vi "Verify Idle.vi"(8 "error in (no error)":errorcluster, 11 "Instrument in":refnum<class "Instrument.lvclass">) -> (0 "error out":errorcluster, 3 "Instrument out":refnum<class "Instrument.lvclass">)   [LabVIEW 2018, in "Instrument.lvclass"]
uses:
  Instrument.lvclass
  Instrument.lvclass/Instrument.ctl
  Device/Optics/Opt_Selector/Opt_Selector.lvclass
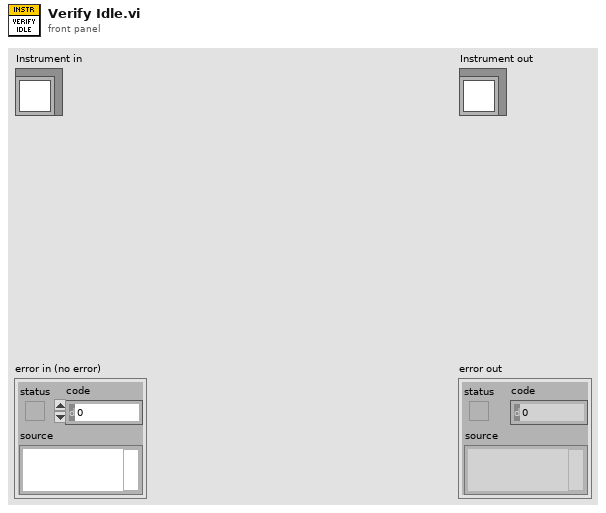
[diagram p1: front panel]
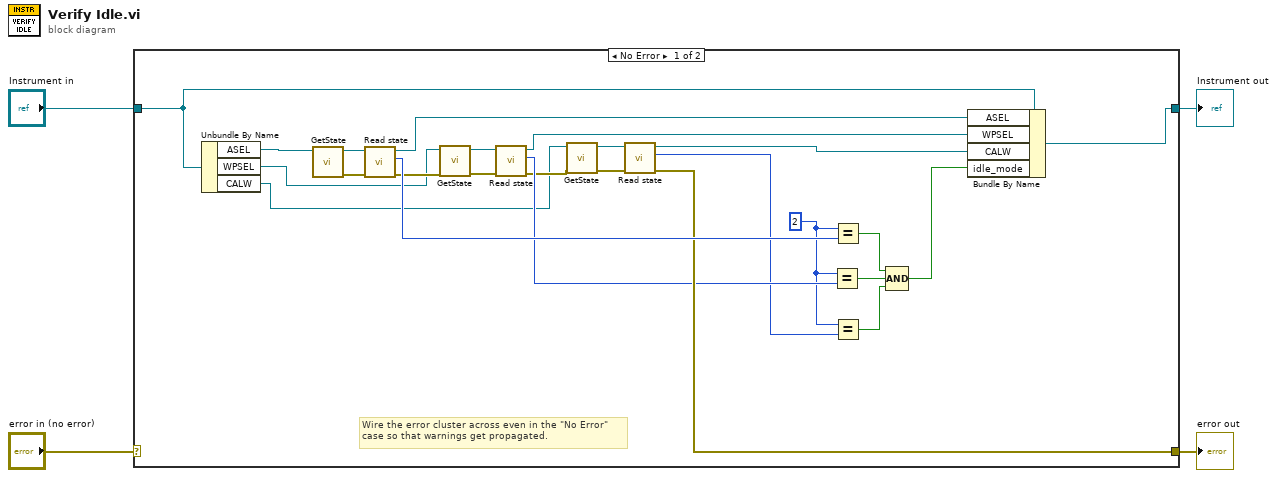
[diagram p0: block diagram]
diagram:
  n1 = case shown="No Error" "error in (no error)" {
    selector: "error in (no error)" -> [_ w31]
    tunnel: [w22 w31] -> w3
    tunnel: [w6 w30] -> w1
    tunnel: "Instrument in" -> [w10 w30]
    frame No Error {
      w19 = 2
      # "Wire the error cluster across even in the \"No Error\"\ncase so that warnings get propagated."
      n2 = Unbundle By Name(w10) -> ("ASEL"=w15:refnum<class "Opt_Selector.lvclass">, "WPSEL"=w12:refnum<class "Opt_Selector.lvclass">, "CALW"=w11:refnum<class "Opt_Selector.lvclass">)
      n3 = call-dynamic "GetState.vi"("Optics in"=w15) -> ("error out"=w28:errorcluster, "Optics out"=w29:refnum<class "Opt_Selector.lvclass">)  [unwired: 9 in]
      n4 = call-dynamic "Read state.vi"("error in (no error)"=w28, "Optics in"=w29) -> ("error out"=w14:errorcluster, "state"=w25:u8, "Optics out"=w9:refnum<class "Opt_Selector.lvclass">)  [unwired: 7 in]
      n5 = call-dynamic "GetState.vi"("error in (no error)"=w14, "Optics in"=w12) -> ("error out"=w26:errorcluster, "Optics out"=w27:refnum<class "Opt_Selector.lvclass">)  [unwired: 8 in]
      n6 = call-dynamic "Read state.vi"("error in (no error)"=w26, "Optics in"=w27) -> ("error out"=w13:errorcluster, "state"=w21:u8, "Optics out"=w8:refnum<class "Opt_Selector.lvclass">)  [unwired: 7 in]
      n7 = call-dynamic "GetState.vi"("error in (no error)"=w13, "Optics in"=w11) -> ("error out"=w23:errorcluster, "Optics out"=w24:refnum<class "Opt_Selector.lvclass">)  [unwired: 8 in]
      n8 = call-dynamic "Read state.vi"("error in (no error)"=w23, "Optics in"=w24) -> ("error out"=w22:errorcluster, "state"=w20:u8, "Optics out"=w7:refnum<class "Opt_Selector.lvclass">)  [unwired: 7 in]
      n9 = Equal?(x=w19, y=w21) -> (x = y?=w17:bool)
      n10 = Equal?(x=w19, y=w25) -> (x = y?=w18:bool)
      n11 = Equal?(x=w19, y=w20) -> (x = y?=w16:bool)
      n12 = Compound Arithmetic op=AND(w18, w17, w16) -> (w5:bool)
      n13 = Bundle By Name(cluster=w10, "ASEL"=w9, "WPSEL"=w8, "CALW"=w7, "idle_mode"=w5) -> (w6:refnum<class "Instrument.lvclass">)
    }
    frame Error {
    }
  }
  "error out" <- w3
  "Instrument out" <- w1
